vi "Byte Buffer.Write (I16).vi"(8 "error in (no error)":errorcluster, 9 "value":i16, 10 "buffer offset":i32, 11 "Byte Buffer in":refnum<class "Byte Buffer.lvclass">) -> (0 "error out":errorcluster, 3 "Byte Buffer out":refnum<class "Byte Buffer.lvclass">)   [LabVIEW 2016, in "VeriStand Data.lvlib" / "Byte Buffer.lvclass"]
doc: "Writes <B>value</B> to the provided <B>Byte Buffer</B> at location <B>buffer offset</B> in the format of the data type specified."
uses:
  Byte Buffer.lvclass
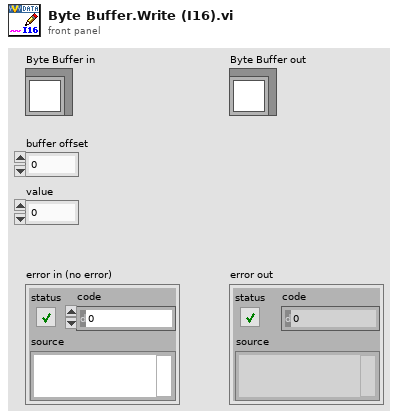
[diagram p1: front panel]
types:
  T1 = enum16{"big-endian, network order", "native, host order", "little-endian"}
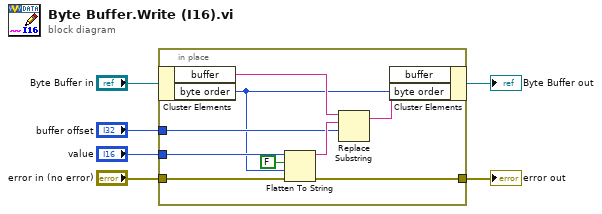
[diagram p0: block diagram]
diagram:
  n1 = in-place {
    in-place-border: "value" -> [w15]
    in-place-border: "buffer offset" -> [w8]
    in-place-border: [w12] -> w4
    in-place-border: "error in (no error)" -> [w11]
    n2 = in-place-cluster #1("Byte Buffer in") -> ("buffer"=w10:string, "byte order"=w7:T1)
    n3 = Flatten To String(anything=w15, prepend array or string size? (T)=FALSE, byte order (0:big-endian, network order)=w7, error in (no error)=w11) -> (data string=w13:string, error out=w12:errorcluster)  [unwired: 1 out]
    n4 = Replace Substring(3:w8, 4:w13, 5:w10) -> (1:w9:string)  [unwired: 1 in, 1 out]
    n5 = in-place-cluster #1("buffer"=w9, "byte order"=w7) -> (→"Byte Buffer out":refnum<class "Byte Buffer.lvclass">)
  }
  "error out" <- w4
